vi "TestStand.ValidateVariableName.vi"(8 "error in":errorcluster, 11 "Name":string) -> (0 "error out":errorcluster, 3 "Valid?":bool)   [LabVIEW 2019, in "Tools.lvlib"]
doc: "This VI checks whether <b>Name</b> is a valid string that can be used as a variable name in TestStand."
uses:
  <vilib>/regexp/Match Regular Expression.xnode
  Tools.lvlib
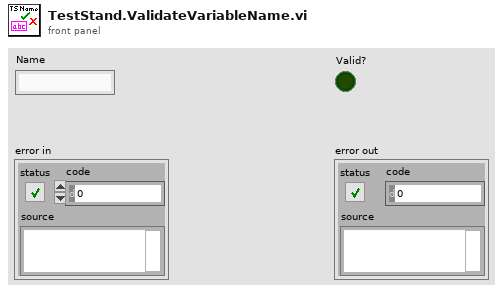
[diagram p1: front panel]
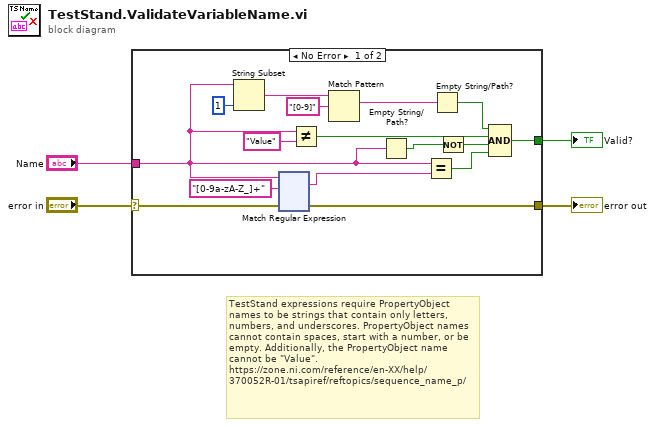
[diagram p0: block diagram]
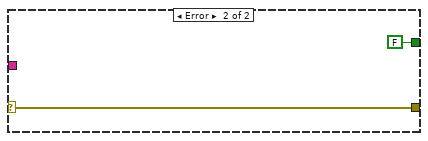
[diagram p2: hidden frame]
diagram:
  # "TestStand expressions require PropertyObject names to be strings that contain only letters, numbers, and underscores. PropertyObject names cannot contain spaces, start with a number, or be empty. Additionally, the PropertyObject name cannot be \"Value\".\nhttps://zone.ni.com/reference/en-XX/help/370052R-01/tsapiref/reftopics/sequence_name_p/"
  n1 = case shown="No Error" "error in" {
    selector: "error in" -> [w13 w135]
    tunnel: "Name" -> [w7 _]
    tunnel: [w15 FALSE] -> w3
    tunnel: [w14 w135] -> w2
    frame No Error {
      n2 = String Subset(string=w7, length (rest)=1 ("length (rest)")) -> (substring=w18:string)  [unwired: 1 in]
      n3 = xnode "Match Regular Expression"("input string"=w7, "regular expression"="[0-9a-zA-Z_]+", "error in"=w13) -> ("whole match"=w20:string, "error out"=w14:errorcluster)  [unwired: 3 in, 3 out]
      n4 = Not Equal?(x=w7, y="Value") -> (x != y?=w10:bool)
      n5 = Match Pattern(string=w18, regular expression="[0-9]") -> (match substring=w16:string)  [unwired: 1 in, 3 out]
      n6 = Empty String/Path?(string/path=w7) -> (empty?=w6:bool)
      n7 = Equal?(x=w7, y=w20) -> (x = y?=w8:bool)
      n8 = Empty String/Path?(string/path=w16) -> (empty?=w11:bool)
      n9 = Not(x=w6) -> (.not. x?=w5:bool)
      n10 = Compound Arithmetic op=AND(w11, w10, w5, w8) -> (w15:bool)
    }
    frame Error {
    }
  }
  "Valid?" <- w3
  "error out" <- w2
